vi "Sequence Data to Sytem CMDs.vi"(9 "Remaining Match Time":dbl, 11 "Sequence Data":T5 {"Auto Angle" scale format="%.3f"}) -> (0 "CMD_ACT_Wrist_Data Out":T1, 1 "CMD_ACT_Grabber_Data Out":T19, 2 "CMD_ACT_Shooter_Data Out":T17={"Mode"=enum."STOP", "Position (counts)"=0, "Velocity (0-1)"=1.0}, 3 "CMD_ACT_Drive_Data Out":T10 {"Auto Angle" scale format="%.3f"; "Direction"."Rotate(Yaw) CCW 1 CW -1" scale=1.0..-1.0; "Direction"."Traverse"."Angle" scale format="%.3f"; "Direction"."Traverse"."Velocity" scale=-1.0..1.0 scale format="%.1f"}, 4 "CMD_ACT_Extend Out":T3, 5 "Max Wait Time Out":dbl)   [LabVIEW 2020, in "2023-Auto_CMD.lvlib"]
uses:
  2023-Auto_CMD.lvlib
  Grabber/Cluster_CMD_ACT_Data.ctl
  Shared Code/TypeDefs/ENUM_Grabber_CMD_Mode Select.ctl
  Sholder/Cluster_CMD_ACT_Data.ctl
  Shared Code/TypeDefs/ENUM_Sholder_CMD_Mode Select.ctl
  SwerveDrive/Cluster_CMD_ACT_Data.ctl
  Shared Code/TypeDefs/ENUM_Swerve_CMD_Mode Select.ctl
  Shared Code/TypeDefs/Cluster_CMD_Direction Data.ctl
  Shared Code/TypeDefs/Cluster_Module Velocity-Direction-Rotations.ctl
  Shared Code/TypeDefs/Level_Velocity plus-minus 1.ctl
  Shared Code/TypeDefs/Dial_Compase heading unit circle CCW positive.ctl
  Type Defs/NUM_Rotate Input.ctl
  Shared Code/TypeDefs/Cluster_X-Y.ctl
  Shared Code/TypeDefs/Cluster_Auto Sequence Settings.ctl
  ENUM_Drive Mode Select.ctl
  MotionMaser/ENUM_Pose List.ctl
  Extention/Cluster_CMD_ACT_Data.ctl
  Shared Code/TypeDefs/ENUM_Extend_CMD_Mode Select.ctl
  Wrist/Cluster_CMD_ACT_Data.ctl
  Shared Code/TypeDefs/ENUM_Wrist_CMD_Mode Select.ctl
  Grabber/Grabber_ACT.lvlib
  Sholder/Sholder_ACT.lvlib
  SwerveDrive/SwerveDrive_ACT.lvlib
  Extention/Extend_ACT.lvlib
  Wrist/Wrist_ACT.lvlib
  MotionMaser/MotionMaster_SubCMD.lvlib
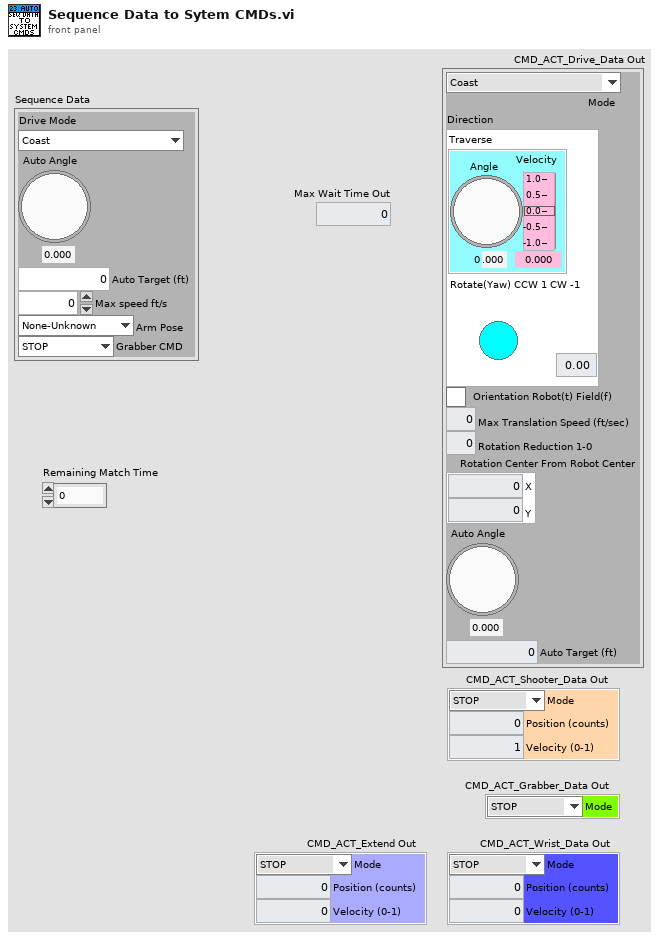
[diagram p1: front panel]
types:
  T1 = typedef "Wrist_ACT.lvlib/Cluster_CMD_ACT_Data.ctl" = cluster{"Mode":T2, "Position (counts)":i32, "Velocity (0-1)":dbl}
  T2 = typedef "ENUM_Wrist_CMD_Mode Select.ctl" = enum16{"STOP", "Position", "Speed"}
  T3 = typedef "Extend_ACT.lvlib/Cluster_CMD_ACT_Data.ctl" = cluster{"Mode":T4, "Position (counts)":i32, "Velocity (0-1)":dbl}
  T4 = typedef "ENUM_Extend_CMD_Mode Select.ctl" = enum16{"STOP", "Position", "Velocity", "Force Home"}
  T5 = typedef "Cluster_Auto Sequence Settings.ctl" = cluster{"Drive Mode":T6, "Auto Angle":T7, "Auto Target (ft)":dbl, "Max speed ft/s":dbl, "Arm Pose ":T8, "Grabber CMD":T9}
  T6 = typedef "2023-Auto_CMD.lvlib/ENUM_Drive Mode Select.ctl" = enum16{"Coast", "To Position", "Rotation Absolute", "Balance on Charger", "Brake", "Lock"}
  T7 = typedef "Dial_Compase heading unit circle CCW positive.ctl" = dbl
  T8 = typedef "MotionMaster_SubCMD.lvlib/ENUM_Pose List.ctl" = enum16{"None-Unknown", "Intake", "Score High", "Score Mid", "Safe Position", "Home Pos"}
  T9 = typedef "ENUM_Grabber_CMD_Mode Select.ctl" = enum16{"STOP", "Intake", "Eject"}
  T10 = typedef "SwerveDrive_ACT.lvlib/Cluster_CMD_ACT_Data.ctl" = cluster{"Mode":T11, "Direction":T12, "Orientation Robot(t) Field(f)":bool, "Max Translation Speed (ft/sec)":dbl, "Rotation Reduction 1-0":dbl, "Rotation Center From Robot Center":T16, "Auto Angle":T7, "Auto Target (ft)":dbl}
  T11 = typedef "ENUM_Swerve_CMD_Mode Select.ctl" = enum16{"Coast", "Manual", "Auto Trans Auto Rotate", "Manual Trans Auto Rotate", "Balance", "Stop Brake", "Lock Wheels"}
  T12 = typedef "Cluster_CMD_Direction Data.ctl" = cluster{"Traverse":T13, "Rotate(Yaw) CCW 1 CW -1":T15}
  T13 = typedef "Cluster_Module Velocity-Direction-Rotations.ctl" = cluster{"Velocity":T14, "Angle":T7, "Rotations Count":dbl}
  T14 = typedef "Level_Velocity plus-minus 1.ctl" = dbl
  T15 = typedef "NUM_Rotate Input.ctl" = dbl
  T16 = typedef "Cluster_X-Y.ctl" = cluster{"X":dbl, "Y":dbl}
  T17 = typedef "Sholder_ACT.lvlib/Cluster_CMD_ACT_Data.ctl" = cluster{"Mode":T18, "Position (counts)":i32, "Velocity (0-1)":dbl}
  T18 = typedef "ENUM_Sholder_CMD_Mode Select.ctl" = enum16{"STOP", "Position", "Percent out"}
  T19 = typedef "Grabber_ACT.lvlib/Cluster_CMD_ACT_Data.ctl" = cluster{"Mode":T9}
  T20 = typedef "Cluster_Pose Positions.ctl" = cluster{"Sholder":i32, "Extend":i32, "Wrist":i32}
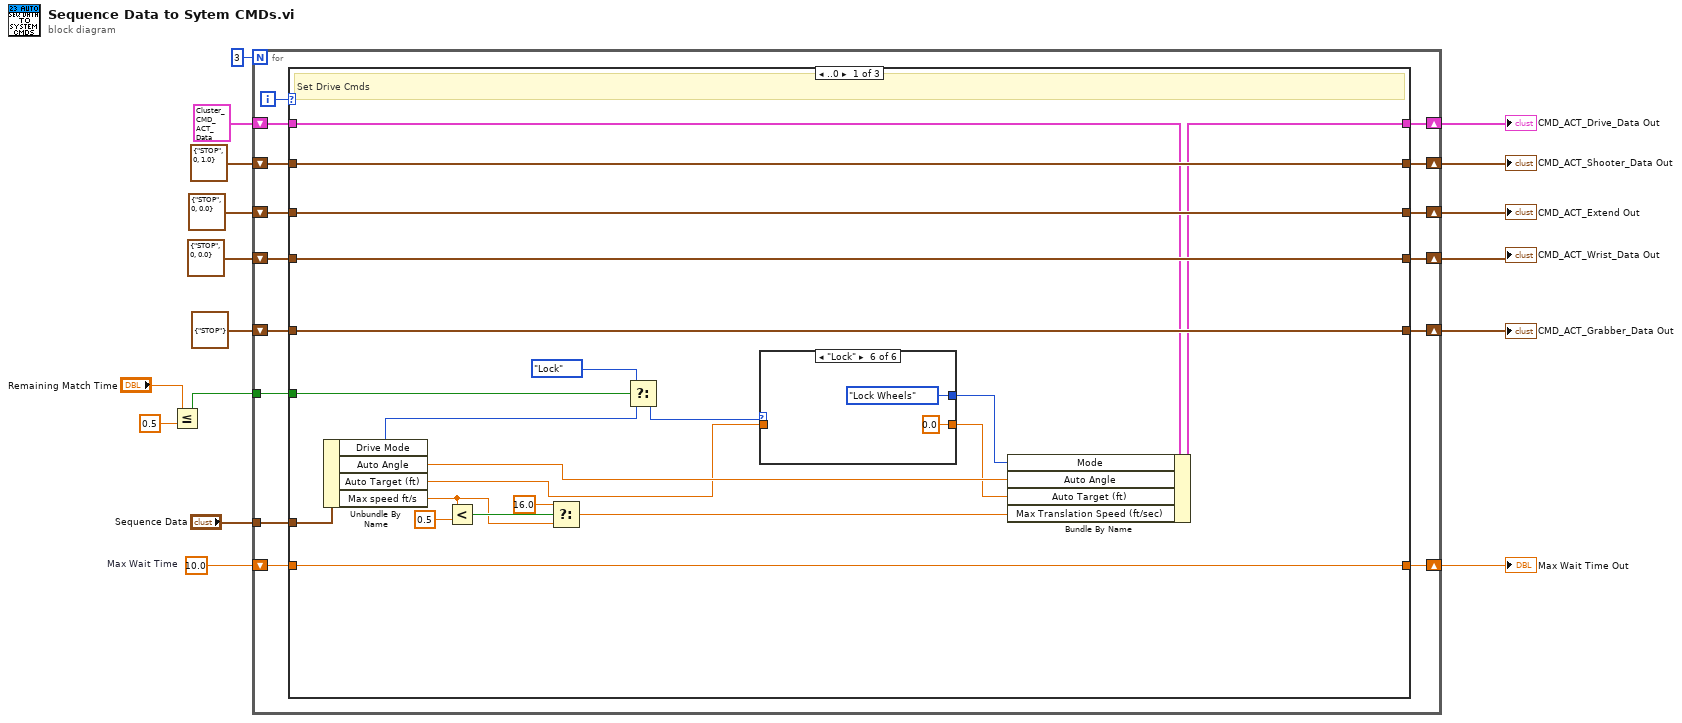
[diagram p0: block diagram]
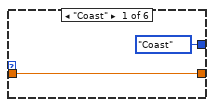
[diagram p2: hidden frame]
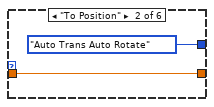
[diagram p3: hidden frame]
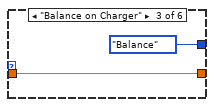
[diagram p4: hidden frame]
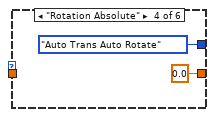
[diagram p5: hidden frame]
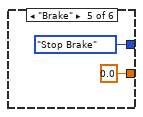
[diagram p6: hidden frame]
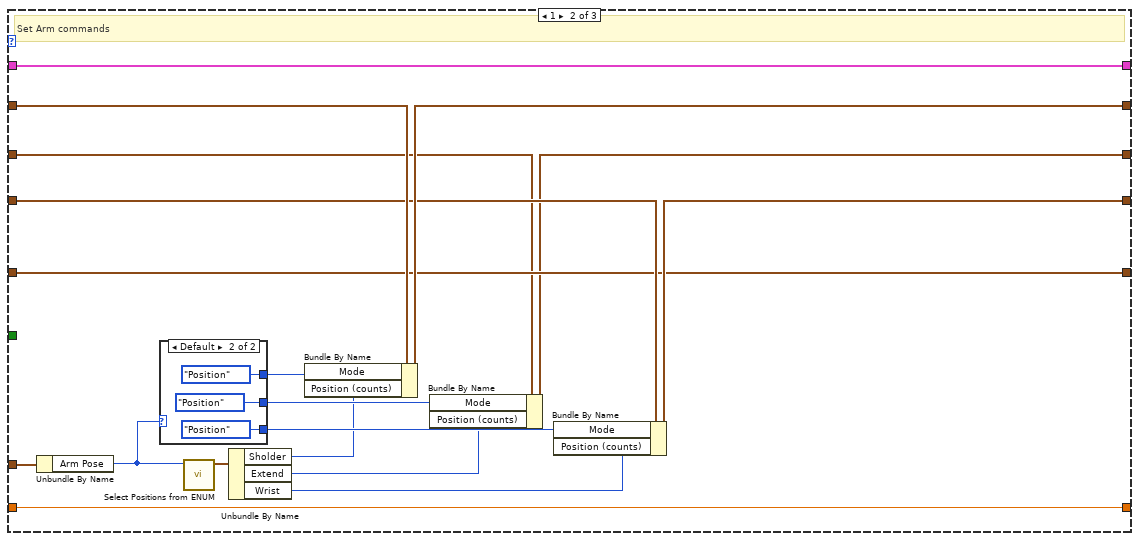
[diagram p7: hidden frame]
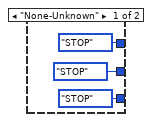
[diagram p8: hidden frame]
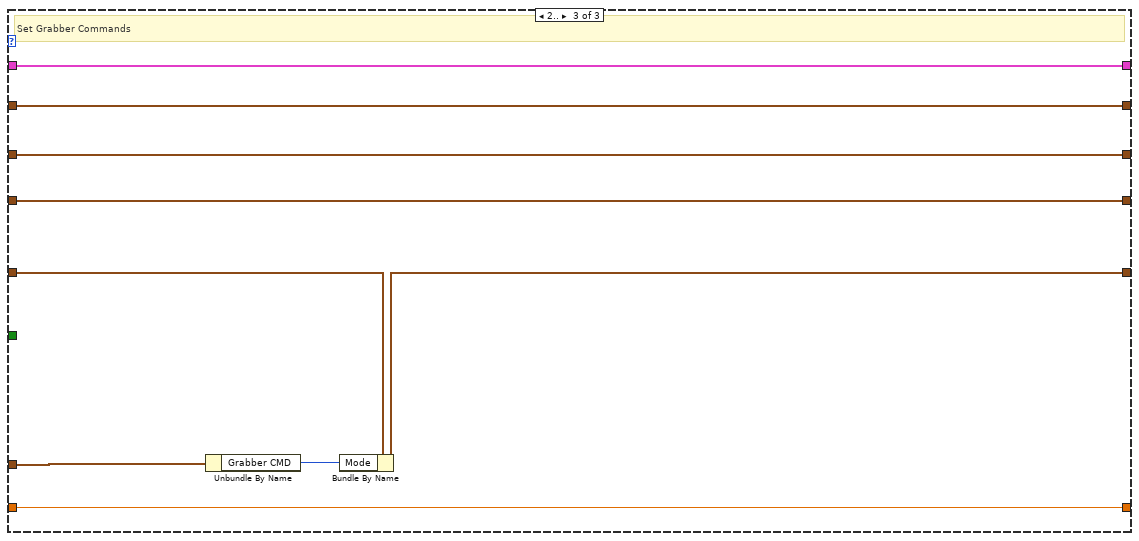
[diagram p9: hidden frame]
diagram:
  w14 = 10.0  # Max Wait Time
  n1 = Less Or Equal?(x="Remaining Match Time", y=0.5) -> (x <= y?=w1:bool)
  n2 = for {
    N: 3 -> [_]
    tunnel: "Sequence Data" -> [w25]
    shift-right: [w26] -> w10
    shift-left: T10 {"Mode"=enum."Coast", "Direction"={"Traverse"={"Velocity"=0.0, "Angle"=0.0, "Rotations Count"=0.0}, "Rotate(Yaw) CCW 1 CW -1"=0.0}, "Orientation Robot(t) Field(f)"=FALSE, "Max Translation Speed (ft/sec)"=0.0, "Rotation Reduction 1-0"=0.0, "Rotation Center From Robot Center"={"X"=0.0, "Y"=0.0}, "Auto Angle"=0.0, "Auto Target (ft)"=0.0} ("CMD_ACT_Drive_Data Out") -> [w31]
    shift-right: [w27] -> w16
    shift-left: T17 {"Mode"=enum."STOP", "Position (counts)"=0, "Velocity (0-1)"=1.0} ("CMD_ACT_Shooter_Data Out") -> [w30]
    shift-right: [w28] -> w17
    shift-left: T19 {"Mode"=enum."STOP"} ("CMD_ACT_Grabber_Data Out") -> [w29]
    shift-right: [w23] -> w8
    shift-left: T3 {"Mode"=enum."STOP", "Position (counts)"=0, "Velocity (0-1)"=0.0} ("CMD_ACT_Extend Out") -> [w24]
    shift-right: [w21] -> w13
    shift-left: w14 -> [w22]
    shift-right: [w19] -> w5
    shift-left: T1 {"Mode"=enum."STOP", "Position (counts)"=0, "Velocity (0-1)"=0.0} ("CMD_ACT_Template_Data") -> [w20]
    tunnel: w1 -> [w18]
    i -> [w32]
    n3 = case shown="..0" w32 {
      tunnel: w31 -> [w43 w83 w97]
      tunnel: w30 -> [w53 w79 w98]
      tunnel: w29 -> [w50 w74 w91]
      tunnel: [w50 w74 w92] -> w28
      tunnel: [w53 w80 w98] -> w27
      tunnel: [w44 w83 w97] -> w26
      tunnel: w25 -> [w48 w81 w93]
      tunnel: w24 -> [w52 w72 w94]
      tunnel: [w52 w73 w94] -> w23
      tunnel: w22 -> [w51 w82 w96]
      tunnel: [w51 w82 w96] -> w21
      tunnel: w20 -> [w49 w77 w95]
      tunnel: [w49 w78 w95] -> w19
      tunnel: w18 -> [w36 _ _]
      frame ..0 {
        # "Set Drive Cmds"
        n4 = Unbundle By Name(w48) -> ("Drive Mode"=w35:T6, "Auto Angle"=w39:T7, "Auto Target (ft)"=w38:dbl, "Max speed ft/s"=w40:dbl)
        n5 = Less?(x=w40, y=0.5) -> (x < y?=w46:bool)
        n6 = Select(t=16.0, s=w46, f=w40) -> (s? t:f=w41:dbl)
        n7 = Select(t=ENUM_Drive_Mode_Select."Lock", s=w36, f=w35) -> (s? t:f=w34:T6)
        n8 = case shown="\"Lock\"" w34 {
          tunnel: [ENUM_Swerve_CMD_Mode_Select."Coast" ("Mode") ENUM_Swerve_CMD_Mode_Select."Auto Trans Auto Rotate" ("Mode") ENUM_Swerve_CMD_Mode_Select."Balance" ("Mode") ENUM_Swerve_CMD_Mode_Select."Auto Trans Auto Rotate" ("Mode") ENUM_Swerve_CMD_Mode_Select."Stop Brake" ("Mode") ENUM_Swerve_CMD_Mode_Select."Lock Wheels" ("Mode")] -> w42
          tunnel: w38 -> [w54 w56 w58 _ _ _]
          tunnel: [w54 w56 w58 0.0 ("Auto Target (ft)") 0.0 ("Auto Target (ft)") 0.0 ("Auto Target (ft)")] -> w37
          frame "Coast" {
          }
          frame "To Position" {
          }
          frame "Balance on Charger" {
          }
          frame "Rotation Absolute" {
          }
          frame "Brake" {
          }
          frame "Lock" {
          }
        }
        n9 = Bundle By Name(cluster=w43, "Mode"=w42, "Auto Angle"=w39, "Auto Target (ft)"=w37, "Max Translation Speed (ft/sec)"=w41) -> (w44:T10)
      }
      frame 1 {
        # "Set Arm commands"
        n10 = Unbundle By Name(w81) -> ("Arm Pose"=w70:T8)
        n11 = case shown="Default" w70 {
          tunnel: [ENUM_Sholder_CMD_Mode_Select."STOP" ("Mode") ENUM_Sholder_CMD_Mode_Select."Position" ("Mode")] -> w76
          tunnel: [ENUM_Wrist_CMD_Mode_Select."STOP" ("Mode 2") ENUM_Wrist_CMD_Mode_Select."Position" ("Mode 2")] -> w75
          tunnel: [ENUM_Extend_CMD_Mode_Select."STOP" ("Mode") ENUM_Extend_CMD_Mode_Select."Position" ("Mode")] -> w71
          frame "None-Unknown" {
          }
          frame Default {
          }
        }
        n12 = call "Select Positions from ENUM.vi"("Pose"=w70) -> ("Selectet  Position Out"=w69:T20)  [unwired: 10 in]
        n13 = Unbundle By Name(w69) -> ("Sholder"=w68:i32, "Extend"=w67:i32, "Wrist"=w66:i32)
        n14 = Bundle By Name(cluster=w79, "Mode"=w76, "Position (counts)"=w68) -> (w80:T17)
        n15 = Bundle By Name(cluster=w72, "Mode"=w71, "Position (counts)"=w67) -> (w73:T3)
        n16 = Bundle By Name(cluster=w77, "Mode"=w75, "Position (counts)"=w66) -> (w78:T1)
      }
      frame 2.. {
        # "Set Grabber Commands"
        n17 = Unbundle By Name(w93) -> ("Grabber CMD"=w90:T9)
        n18 = Bundle By Name(cluster=w91, "Mode"=w90) -> (w92:T19)
      }
    }
  }
  "CMD_ACT_Grabber_Data Out" <- w17
  "CMD_ACT_Shooter_Data Out" <- w16
  "CMD_ACT_Drive_Data Out" <- w10
  "CMD_ACT_Extend Out" <- w8
  "Max Wait Time Out" <- w13
  "CMD_ACT_Wrist_Data Out" <- w5
